vi "Z900_navX_Internal_UpdateDevice.vi"(8 "error in (no error)":errorcluster, 10 "Interface TypeDefs":T1 {"I2CDevRef"."Device Address" format="%.0x"}, 11 "navX Device":T7={"Interface"={"Protocol"=enum."SERIAL", "Update Rate (4Hz-100Hz)"=4, "navX Open TypeDef"=variant}, "Notify Packet"=refnum, "Loop VI Refnum"=refnum, "Ready to Close Occurrence Refnum"=refnum} {"Interface"."Update Rate (4Hz-100Hz)" min=4 max=60 step=1}) -> (0 "error out":errorcluster, 2 "Interface TypeDefs":T1 {"I2CDevRef"."Device Address" format="%.0x"}, 3 "navX Device":T7={"Interface"={"Protocol"=enum."SERIAL", "Update Rate (4Hz-100Hz)"=4, "navX Open TypeDef"=variant}, "Notify Packet"=refnum, "Loop VI Refnum"=refnum, "Ready to Close Occurrence Refnum"=refnum} {"Interface"."Update Rate (4Hz-100Hz)" min=4 max=60 step=1})   [LabVIEW 2015, in "Apple Pi Gyro Library.lvlib" / "navX Library v2.lvlib"]
doc: "This navX VI handles updating rate and serial protocol for the navX.\nTHIS VI SHOULD NOT BE CALLED BY THE USER!"
uses:
  navX Library v2.lvlib
  TypeDefs/Z900_navX_DeviceTypeDef.ctl
  TypeDefs/Z900_navX_ProtocolTypeDef.ctl
  TypeDefs/Z900_navX_NotifyPacketTypeDef.ctl
  TypeDefs/Z900_navX_ActionTypeDef.ctl
  TypeDefs/Z900_navX_InterfaceTypeDef.ctl
  <vilib>/Rock Robotics/WPI/SerialPort/WPI_SerialPortRef.ctl
  <vilib>/Rock Robotics/WPI/I2C/WPI_I2CDevRef.ctl
  <vilib>/Rock Robotics/SystemInterfaces/i2clib/i2c_bus.ctl
  <vilib>/Rock Robotics/WPI/SPI/WPI_SPIDevRef.ctl
  <vilib>/Rock Robotics/SystemInterfaces/spilib/spi_bus.ctl
  TypeDefs/navX Open TypeDefs/Z900_navX_OpenTypeDef_Serial.ctl
  NI WPI/WPI_SerialPort_USB.ctl
  TypeDefs/Z900_navX_SerialStreamTypeDef.ctl
  TypeDefs/navX Open TypeDefs/Z900_navX_OpenTypeDef_I2C.ctl
  TypeDefs/Z900_navX_DeviceRegisters.ctl
  TypeDefs/navX Open TypeDefs/Z900_navX_OpenTypeDef_SPI.ctl
  NI WPI/NI WPI Serial USB.lvlib
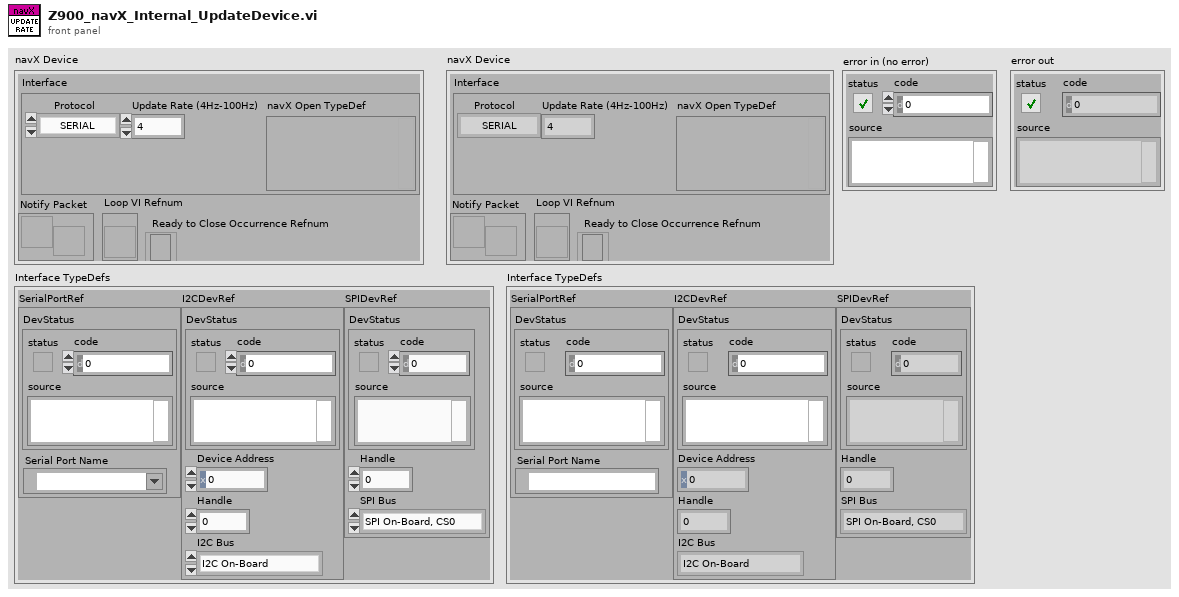
[diagram p1: front panel]
types:
  T1 = typedef "Apple Pi Gyro Library.lvlib/navX Library v2.lvlib/Z900_navX_InterfaceTypeDef.ctl" = cluster{"SerialPortRef":T2, "I2CDevRef":T3, "SPIDevRef":T5}
  T2 = typedef "WPI_SerialPortRef.ctl" = cluster{"DevStatus":errorcluster, "Serial Port Name":refnum<visa-resource-name>}
  T3 = typedef "WPI_I2CDevRef.ctl" = cluster{"DevStatus":errorcluster, "Device Address":u8, "Handle":i32, "I2C Bus":T4}
  T4 = typedef "i2c_bus.ctl" = enum16{"I2C On-Board", "I2C MXP", "Invalid"}
  T5 = typedef "WPI_SPIDevRef.ctl" = cluster{"DevStatus":errorcluster, "Handle":i32, "SPI Bus":T6}
  T6 = typedef "spi_bus.ctl" = enum16{"SPI On-Board, CS0", "SPI On-Board, CS1", "SPI On-Board, CS2", "SPI On-Board, CS3", "SPI MXP", "Invalid"}
  T7 = typedef "Apple Pi Gyro Library.lvlib/navX Library v2.lvlib/Z900_navX_DeviceTypeDef.ctl" = cluster{"Interface":cluster{"Protocol":T8, "Update Rate (4Hz-100Hz)":u8, "navX Open TypeDef":variant}, "Notify Packet":refnum<notifier>, "Loop VI Refnum":refnum<vi>, "Ready to Close Occurrence Refnum":refnum<k4>}
  T8 = typedef "Apple Pi Gyro Library.lvlib/navX Library v2.lvlib/Z900_navX_ProtocolTypeDef.ctl" = enum16{"SERIAL", "I2C", "SPI"}
  T9 = typedef "Apple Pi Gyro Library.lvlib/navX Library v2.lvlib/Z900_navX_OpenTypeDef_Serial.ctl" = cluster{"Serial Port":T10, "Stream Type":T11}
  T10 = typedef "NI WPI Serial USB.lvlib/WPI_SerialPort_USB.ctl" = enum16{"Onboard RS-232", "MXP TTL", "USB"}
  T11 = typedef "Apple Pi Gyro Library.lvlib/navX Library v2.lvlib/Z900_navX_SerialStreamTypeDef.ctl" = enum16{"YRPH", "Quaterinons", "Gyro/Raw", "AHRS", "AHRSAndPositioning"}
  T12 = typedef "Apple Pi Gyro Library.lvlib/navX Library v2.lvlib/Z900_navX_OpenTypeDef_I2C.ctl" = cluster{"I2C Bus":T4}
  T13 = typedef "Apple Pi Gyro Library.lvlib/navX Library v2.lvlib/Z900_navX_OpenTypeDef_SPI.ctl" = cluster{"SPI Bus":T6, "Clock Rate (Hz)":dbl}
  T14 = typedef "Apple Pi Gyro Library.lvlib/navX Library v2.lvlib/Z900_navX_DeviceRegisters.ctl" = u8
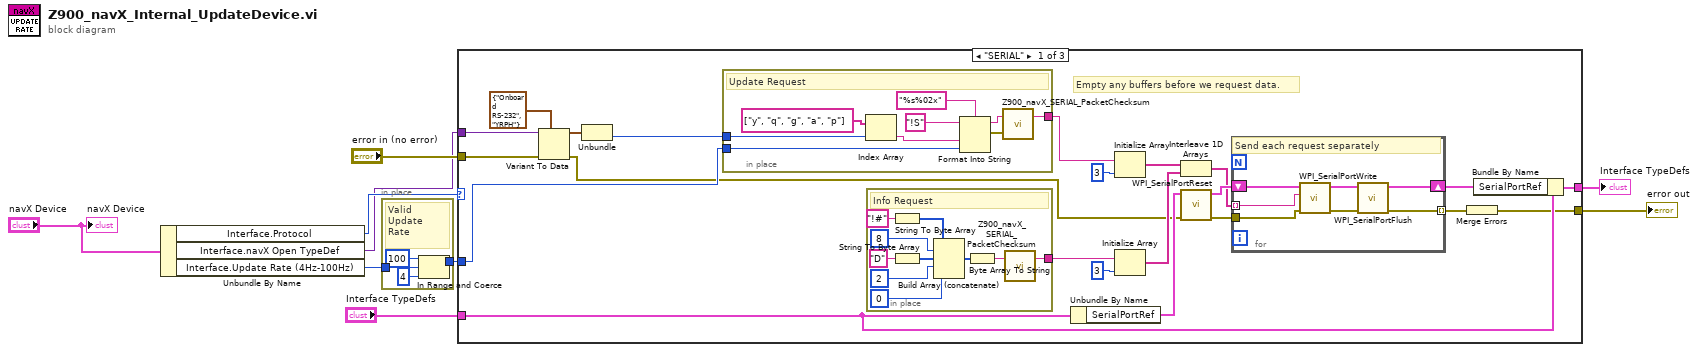
[diagram p0: block diagram]
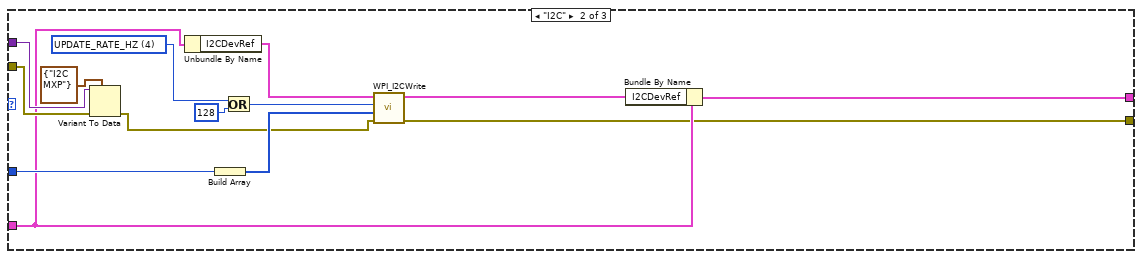
[diagram p2: hidden frame]
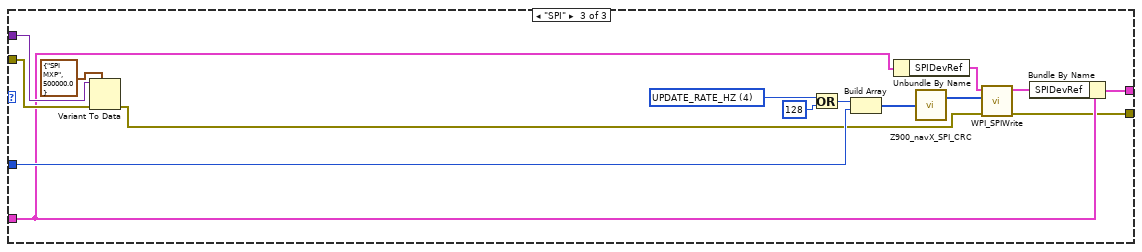
[diagram p3: hidden frame]
diagram:
  n1 = Unbundle By Name("navX Device") -> ("Interface.Protocol"=w8:T8, "Interface.navX Open TypeDef"=w4:variant, "Interface.Update Rate (4Hz-100Hz)"=w3:u8)
  n2 = in-place {
    in-place-border: w3 -> [w13]
    in-place-border: [w10] -> w2
    # "Valid\nUpdate\nRate"
    n3 = In Range and Coerce(upper limit=u8 100, x=w13, lower limit=u8 4) -> (coerced(x)=w10:u8)  [unwired: 1 out]
  }
  n4 = case shown="\"SERIAL\"" w8 {
    tunnel: w4 -> [w35 w75 w90]
    tunnel: "error in (no error)" -> [w33 w73 w88]
    tunnel: "Interface TypeDefs" -> [w30 w66 w80]
    tunnel: w2 -> [w28 w69 w82]
    tunnel: [w29 w64 w78] -> w5
    tunnel: [w15 w62 w76] -> w1
    frame "SERIAL" {
      # "Empty any buffers before we request data."
      n5 = Variant To Data(error in=w33, type=T9 {"Serial Port"=enum."Onboard RS-232", "Stream Type"=enum."YRPH"} ("navX Serial Open"), Variant=w35) -> (data=w32:T9, error out=w14:errorcluster)
      n6 = Unbundle(w32) -> ("Stream Type"=w31:T11)  [unwired: 1 out]
      n7 = in-place {
        in-place-border: w31 -> [w50]
        in-place-border: [w43] -> w23
        in-place-border: w28 -> [w44]
        # "Update Request"
        n8 = Index Array(array=string[] ["y", "q", "g", "a", "p"], index=w50) -> (element=w45:string)
        n9 = Format Into String(format string="%s%02x", initial string="!S", w45, w44) -> (resulting string=w48:string, error out=w49:errorcluster)  [unwired: 1 in]
        n10 = call "Z900_navX_SERIAL_PacketChecksum.vi"("error in (no error)"=w49, "Packet"=w48) -> ("Terminated Packet"=w43:string)  [unwired: 1 out]
      }
      n11 = in-place {
        in-place-border: [w52] -> w21
        # "Info Request"
        n12 = String To Byte Array(string="!#" ("initial string")) -> (unsigned byte array=w59:u8[])
        n13 = String To Byte Array(string="D" ("initial string")) -> (unsigned byte array=w57:u8[])
        n14 = Build Array (concatenate)(w59, 8, w57, 2, 0) -> (w54:i32[])
        n15 = Byte Array To String(unsigned byte array=w54) -> (string=w53:string)
        n16 = call "Z900_navX_SERIAL_PacketChecksum.vi"("Packet"=w53) -> ("Terminated Packet"=w52:string)  [unwired: 1 in, 1 out]
      }
      n17 = Unbundle By Name(w30) -> ("SerialPortRef"=w26:T2)
      n18 = Initialize Array(w23, 3 ("dimension size")) -> (w20:string[])
      n19 = Initialize Array(w21, 3 ("dimension size")) -> (w19:string[])
      n20 = Interleave 1D Arrays(w20, w19) -> (w18:string[])
      n21 = call <vilib>:"WPI_SerialPortReset.vi"("error in (no error)"=w14, "SerialPortRef"=w26) -> ("error out"=w24:errorcluster, "SerialPortRef"=w25:T2)  [unwired: 8 in]
      n22 = for {
        tunnel: w24 -> [w39]
        tunnel: w18 -> [w38] mode=indexing
        shift-right: [w37] -> w17
        shift-left: w25 -> [w40]
        tunnel: [w36] -> w16 mode=indexing
        # "Send each request separately"
        n23 = call <vilib>:"WPI_SerialPortWrite.vi"("error in (no error)"=w39, "Buffer"=w38, "SerialPortRef"=w40) -> ("error out"=w41:errorcluster, "SerialPortRef"=w42:T2)  [unwired: 6 in, 1 out]
        n24 = call <vilib>:"WPI_SerialPortFlush.vi"("error in (no error)"=w41, "SerialPortRef"=w42) -> ("error out"=w36:errorcluster, "SerialPortRef"=w37:T2)  [unwired: 8 in]
      }
      n25 = Merge Errors(w16) -> (w15:errorcluster)
      n26 = Bundle By Name(cluster=w30, "SerialPortRef"=w17) -> (w29:T1)
    }
    frame "I2C" {
      w70 = T14 4 items=["WHOAMI"=0, "HW_REV"=1, "FW_VER_MAJOR"=2, "FW_VER_MINOR"=3, "UPDATE_RATE_HZ"=4, "ACCEL_FSR_G"=5, "GYRO_FSR_DPS"=6, "OP_STATUS"=8, "CAL_STATUS"=9, "SELFTEST_STATUS"=10, "CAPABILITY_FLAGS_L"=11, "CAPABILITY_FLAGS_H"=12, "SENSOR_STATUS"=16, "TIMESTAMP"=18, "YAW"=22, "ROLL"=24, "PITCH"=26, "HEADING"=28, "FUSED_HEADING"=30, "ALTITUDE_I"=32, "ALTITUDE_D"=34, "LINERA_ACC_X"=36, "LINERA_ACC_Y"=38, "LINERA_ACC_Z"=40, "QUAT_W"=42, "QUAT_X"=44, "QUAT_Y"=46, "QUAT_Z"=48, "MPU_TEMP_C"=50, "GYRO_X"=52, "GYRO_Y"=54, "GYRO_Z"=56, "ACC_X"=58, "ACC_Y"=60, "ACC_Z"=62, "MAG_X"=64, "MAG_Y"=66, "MAG_Z"=68, "PRESSURE_I"=70, "PRESSURE_D"=72, "PRESSURE_TEMP"=74, "YAW_OFFSET"=76, "QUAT_OFFSET_W"=78, "QUAT_OFFSET_X"=80, "QUAT_OFFSET_Y"=82, "QUAT_OFFSET_Z"=84, "INTEGRATION_CONTROL"=86, "VELOCITY_X"=88, "VELOCITY_Y"=92, "VELOCITY_Z"=96, "DISPLACMENT_X"=100, "DISPLACMENT_Y"=104, "DISPLACEMENT_Z"=108] ("Device Register")
      n27 = Variant To Data(error in=w73, type=T12 {"I2C Bus"=enum."I2C MXP"} ("navX I2C Open"), Variant=w75) -> (error out=w63:errorcluster)  [unwired: 1 out]
      n28 = Unbundle By Name(w66) -> ("I2CDevRef"=w67:T3)
      n29 = Build Array(w69) -> (w68:u8[])
      n30 = Or(x=w70, y=u8 128) -> (x .or. y?=w72:T14)
      n31 = call <vilib>:"WPI_I2CWrite.vi"("error in (no error)"=w63, "I2CDataToSend"=w68, "I2CRegister"=w72, "I2CDevRef"=w67) -> ("error out"=w62:errorcluster, "I2CDevRef"=w65:T3)  [unwired: 6 in]
      n32 = Bundle By Name(cluster=w66, "I2CDevRef"=w65) -> (w64:T1)
    }
    frame "SPI" {
      w84 = T14 4 items=["WHOAMI"=0, "HW_REV"=1, "FW_VER_MAJOR"=2, "FW_VER_MINOR"=3, "UPDATE_RATE_HZ"=4, "ACCEL_FSR_G"=5, "GYRO_FSR_DPS"=6, "OP_STATUS"=8, "CAL_STATUS"=9, "SELFTEST_STATUS"=10, "CAPABILITY_FLAGS_L"=11, "CAPABILITY_FLAGS_H"=12, "SENSOR_STATUS"=16, "TIMESTAMP"=18, "YAW"=22, "ROLL"=24, "PITCH"=26, "HEADING"=28, "FUSED_HEADING"=30, "ALTITUDE_I"=32, "ALTITUDE_D"=34, "LINERA_ACC_X"=36, "LINERA_ACC_Y"=38, "LINERA_ACC_Z"=40, "QUAT_W"=42, "QUAT_X"=44, "QUAT_Y"=46, "QUAT_Z"=48, "MPU_TEMP_C"=50, "GYRO_X"=52, "GYRO_Y"=54, "GYRO_Z"=56, "ACC_X"=58, "ACC_Y"=60, "ACC_Z"=62, "MAG_X"=64, "MAG_Y"=66, "MAG_Z"=68, "PRESSURE_I"=70, "PRESSURE_D"=72, "PRESSURE_TEMP"=74, "YAW_OFFSET"=76, "QUAT_OFFSET_W"=78, "QUAT_OFFSET_X"=80, "QUAT_OFFSET_Y"=82, "QUAT_OFFSET_Z"=84, "INTEGRATION_CONTROL"=86, "VELOCITY_X"=88, "VELOCITY_Y"=92, "VELOCITY_Z"=96, "DISPLACMENT_X"=100, "DISPLACMENT_Y"=104, "DISPLACEMENT_Z"=108] ("Device Register")
      n33 = Variant To Data(error in=w88, type=T13 {"SPI Bus"=enum."SPI MXP", "Clock Rate (Hz)"=500000.0} ("navX SPI Open"), Variant=w90) -> (error out=w77:errorcluster)  [unwired: 1 out]
      n34 = Or(x=w84, y=u8 128) -> (x .or. y?=w85:T14)
      n35 = Build Array(w85, w82) -> (w86:T14[])
      n36 = Unbundle By Name(w80) -> ("SPIDevRef"=w81:T5)
      n37 = call "Z900_navX_SPI_CRC.vi"("Message"=w86) -> ("Message with CRC"=w87:u8[])  [unwired: 1 out]
      n38 = call <vilib>:"WPI_SPIWrite.vi"("error in (no error)"=w77, "Data To Send"=w87, "SPIDevRef"=w81) -> ("error out"=w76:errorcluster, "SPIDevRef"=w79:T5)  [unwired: 6 in, 1 out]
      n39 = Bundle By Name(cluster=w80, "SPIDevRef"=w79) -> (w78:T1)
    }
  }
  "error out" <- w1
  "Interface TypeDefs" <- w5
  "navX Device" <- "navX Device"
